vi "DPW Density of Pure Water (Kg to m3).vi"(1 "Pure Water Temprature":dbl[unit]) -> (0 "DPW":dbl[unit])   [LabVIEW 2018]
panel:
  out "Pure Water Temprature":dbl[unit](slide) scale=0.0..100.0
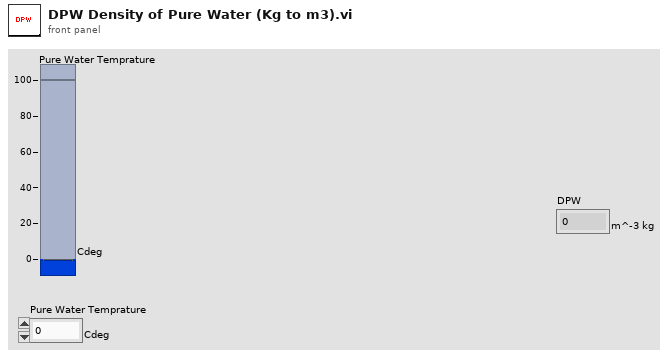
[diagram p1: front panel]
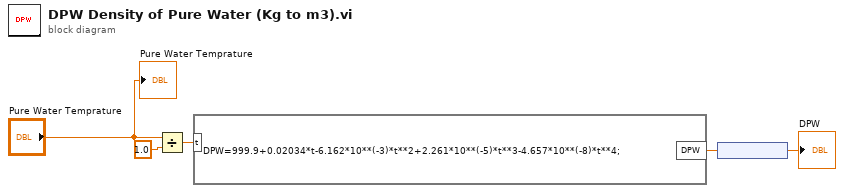
[diagram p0: block diagram]
diagram:
  n1 = Divide(x="Pure Water Temprature", y=dbl[unit] 1.0) -> (x/y=w5:dbl)
  n2 = formula code="DPW=999.9+0.02034*t-6.162*10**(-3)*t**2+2.261*10**(-5)*t**3-4.657*10**(-8)*t**4;"("t"=w5) -> ("DPW"=w1:dbl)
  n3 = node(w1) -> (→"DPW":dbl[unit])
  "Pure Water Temprature" <- "Pure Water Temprature"
